vi "Set Drive Modes.vi"   [LabVIEW 2016]
uses:
  Drive Control Type.ctl
  <vilib>/Rock Robotics/WPI/DriverStation/WPI_DriverStationRobotMode2.ctl
  Drive Globals.vi
  Rotation/Rotation Globals.vi
  Intake/Intake Globals.vi
  Robot Global Data.vi
types:
  T1 = typedef "WPI_DriverStationRobotMode2.ctl" = enum16{"Autonomous Disabled", "Autonomous Enabled", "Teleop Disabled", "Teleop Enabled", "Disconnected", "Finish", "Test Disabled", "Test Enabled", "Emergency Stopped"}
  T2 = typedef "Drive Control Type.ctl" = enum16{"No Op", "Fieldcentric", "Robotcentric", "Reset Wheel Position", "Reset Gyro Value", "Turn to Angle", "Drive For Time"}
  T3 = typedef "Drive Notifier.ctl" = cluster{"Parameter 1":dbl, "Parameter 2":dbl, "Parameter 3":dbl, "Drive Control List":T2, "Parameter 4":dbl, "Gear Angle":dbl, "Parameter 6":dbl, "Parameter 7":dbl, "Parameter 8":dbl, "Parameter 9":dbl, "Robotcentric":bool, "Reset Gyro":bool, "Reset Wheels":bool, "Turn to Gear Left":bool, "Turn to Gear Center":bool, "Turn to Gear Right":bool, "Half Power":bool, "Drive Notifier":refnum<notifier>, "Step":i32}
  T4 = typedef "Rotation Notifier.ctl" = cluster{"Up":bool, "Down":bool, "Rotation Control List":T5, "Control Down":bool, "Manual":bool, "Parameter 1":dbl, "Parameter 2":dbl, "Rotation Notifier":refnum<notifier>, "Step":i32}
  T5 = typedef "Rotation Control Type.ctl" = enum16{"No Op", "Up", "Down", "Control Up", "Control Down"}
  T6 = typedef "Intake Notifier.ctl" = cluster{"In":bool, "Out":bool, "Intake Control List":T7, "Parameter 1":dbl, "Parameter 2":dbl, "Intake Notifier":refnum<notifier>, "Step":i32}
  T7 = typedef "Intake Control Type.ctl" = enum16{"No Op", "In", "Out"}
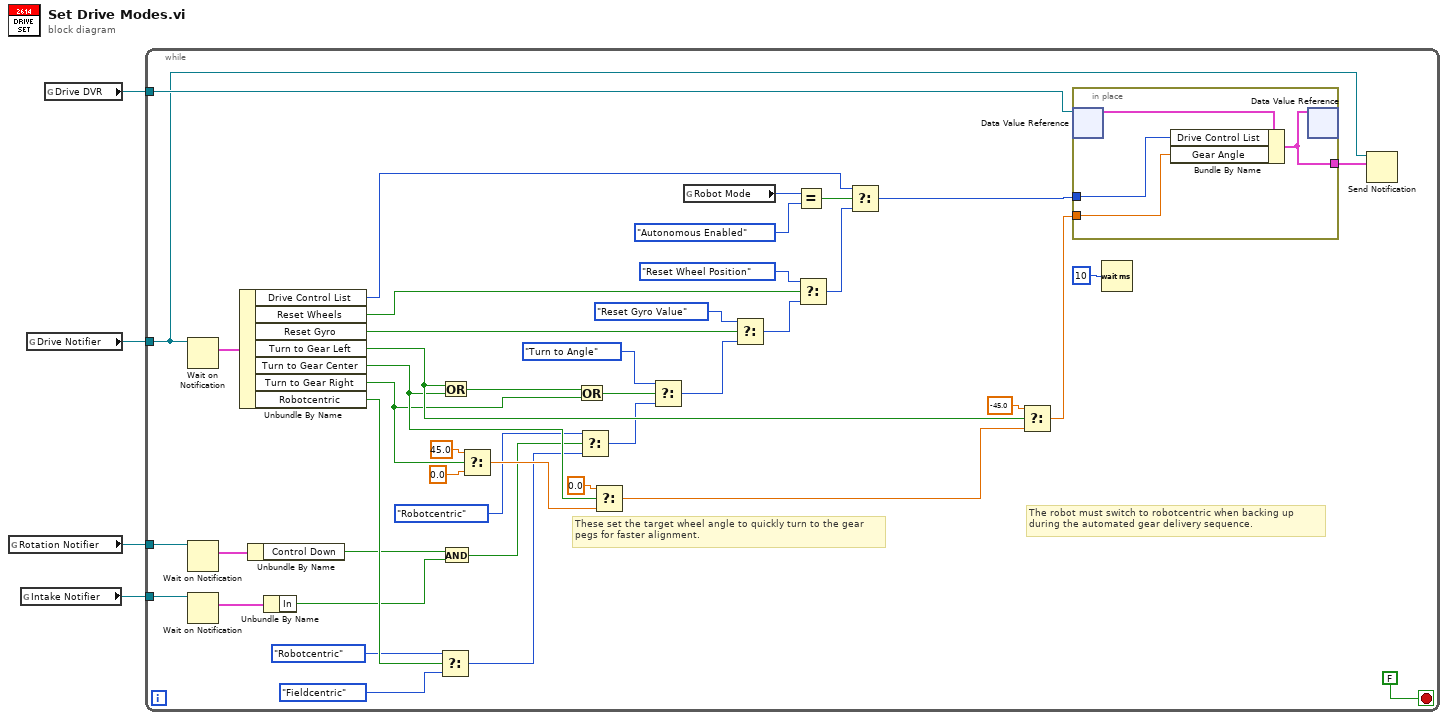
[diagram p0: block diagram]
diagram:
  n1 = global read "Rotation Globals.vi" "Rotation Notifier"() -> (w2:refnum<notifier>)
  n2 = global read "Intake Globals.vi" "Intake Notifier"() -> (w1:refnum<notifier>)
  n3 = global read "Drive Globals.vi" "Drive Notifier"() -> (w3:refnum<notifier>)
  n4 = global read "Drive Globals.vi" "Drive DVR"() -> (w4:refnum<data-value>)
  n5 = while {
    tunnel: w4 -> [w46]
    tunnel: w3 -> [w5]
    tunnel: w2 -> [w21]
    tunnel: w1 -> [w16]
    stop <- FALSE stop-if-true
    # "The robot must switch to robotcentric when backing up\nduring the automated gear delivery sequence."
    # "These set the target wheel angle to quickly turn to the gear\npegs for faster alignment."
    n6 = Wait on Notification(notifier=w5) -> (notification=w44:T3)  [unwired: 3 in, 3 out]
    n7 = Wait on Notification(notifier=w21) -> (notification=w20:T4)  [unwired: 3 in, 3 out]
    n8 = Wait on Notification(notifier=w16) -> (notification=w15:T6)  [unwired: 3 in, 3 out]
    n9 = Unbundle By Name(w44) -> ("Drive Control List"=w6:T2, "Reset Wheels"=w43:bool, "Reset Gyro"=w41:bool, "Turn to Gear Left"=w25:bool, "Turn to Gear Center"=w24:bool, "Turn to Gear Right"=w23:bool, "Robotcentric"=w38:bool)
    n10 = Unbundle By Name(w20) -> ("Control Down"=w14:bool)
    n11 = Unbundle By Name(w15) -> ("In"=w13:bool)
    n12 = Select(t=Drive_Control_Type."Robotcentric" ("Drive Control List"), s=w38, f=Drive_Control_Type."Fieldcentric" ("Drive Control List")) -> (s? t:f=w19:T2)
    n13 = Or(x=w25, y=w24) -> (x .or. y?=w33:bool)
    n14 = And(x=w14, y=w13) -> (x .and. y?=w12:bool)
    n15 = Select(t=45.0, s=w23, f=0.0) -> (s? t:f=w31:dbl)
    n16 = Or(x=w33, y=w23) -> (x .or. y?=w34:bool)
    n17 = Select(t=Drive_Control_Type."Robotcentric" ("Drive Control List"), s=w12, f=w19) -> (s? t:f=w18:T2)
    n18 = Select(t=0.0, s=w24, f=w31) -> (s? t:f=w32:dbl)
    n19 = Select(t=Drive_Control_Type."Turn to Angle" ("Drive Control List"), s=w34, f=w18) -> (s? t:f=w35:T2)
    n20 = global read "Robot Global Data.vi" "Robot Mode"() -> (w11:T1)
    n21 = Select(t=Drive_Control_Type."Reset Gyro Value" ("Drive Control List"), s=w41, f=w35) -> (s? t:f=w39:T2)
    n22 = Equal?(x=w11, y=WPI_DriverStationRobotMode2."Autonomous Enabled") -> (x = y?=w7:bool)
    n23 = Select(t=Drive_Control_Type."Reset Wheel Position" ("Drive Control List"), s=w43, f=w39) -> (s? t:f=w9:T2)
    n24 = Select(t=w6, s=w7, f=w9) -> (s? t:f=w8:T2)
    n25 = Select(t=-45.0, s=w25, f=w32) -> (s? t:f=w30:dbl)
    n26 = in-place {
      in-place-border: w8 -> [w50]
      in-place-border: [w51] -> w45
      in-place-border: w30 -> [w49]
      n27 = in-place-dvr #1(w46) -> (w52:T3)  [unwired: 1 out]
      n28 = Bundle By Name(cluster=w52, "Drive Control List"=w50, "Gear Angle"=w49) -> (w51:T3)
      n29 = in-place-dvr #1(w51) -> ()  [unwired: 2 out]
    }
    n30 = Wait (ms)(milliseconds to wait=u32 10) -> ()  [unwired: 1 out]
    n31 = Send Notification(notification=w45, notifier=w5) -> ()  [unwired: 1 in, 2 out]
  }
